vi "User data_MClr.vi"(0 "Inspector":string="ID-0", 1 "Station":string="EQD", 2 "Vendor":string="Icon", 3 "Number":string="?", 4 "PO#":string="?", 5 "Error In":errorcluster, 6 "base path":path=path "C:/", 8 "prompt (Create Folder)":string="logsController", 10 "file name":string) -> (14 "refnum out":refnum<file>, 19 "error out":errorcluster)   [LabVIEW 2018]
uses:
  Global textParse.vi
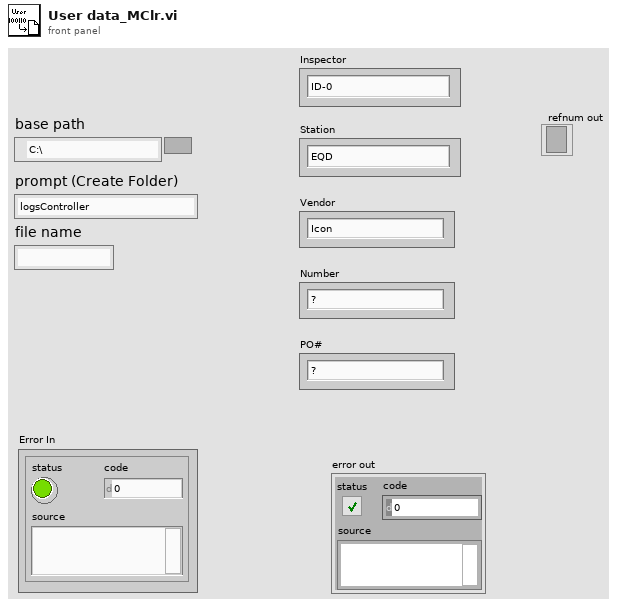
[diagram p1: front panel]
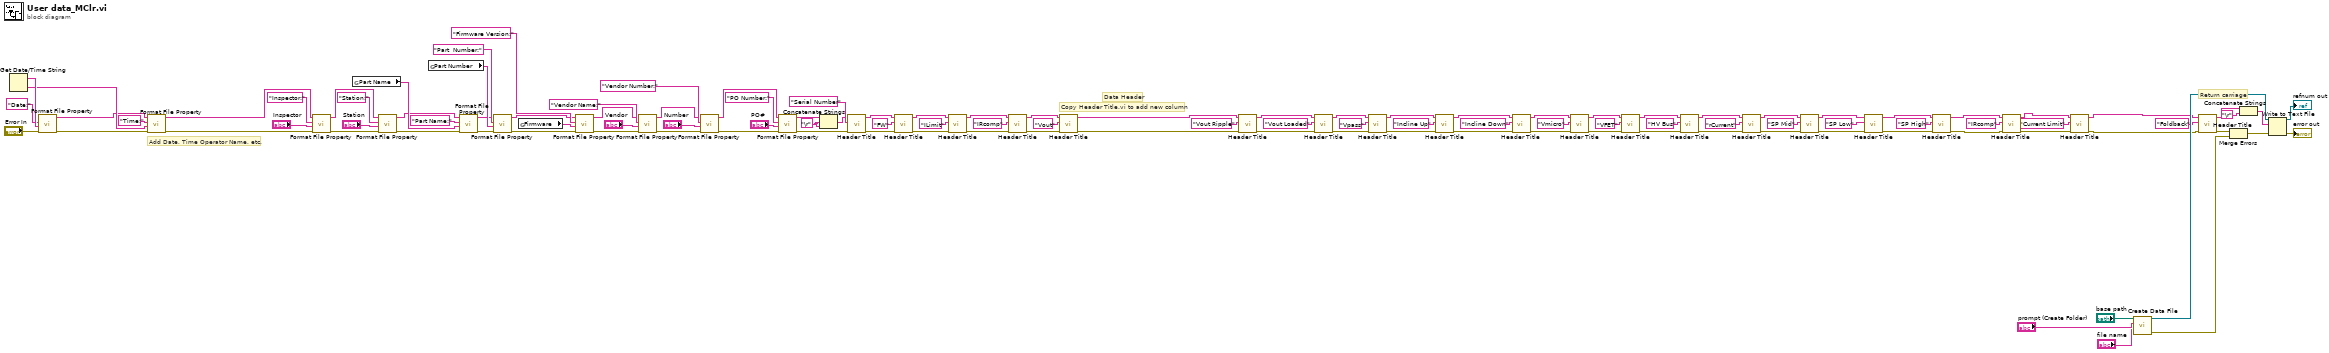
[diagram p0: block diagram]
diagram:
  w74 = "\r"
  # "Return carriage"
  # "Copy Header Title.vi to add new column"
  # "Data Header"
  # "Add Date, Time Operator Name, etc."
  n1 = Get Date/Time String() -> (date string=w110:string, time string=w101:string)  [unwired: 3 in]
  n2 = call "Format File Property.vi"("Error In"="Error In", "File Property Value"=w110, "File Property Name"="Date:") -> ("Error Out"=w108:errorcluster, "String out"=w36:string)  [unwired: 7 in]
  n3 = call "Format File Property.vi"("Error In"=w108, "File Property Value"=w101, "File Property Name"="Time:", "String in"=w36) -> ("Error Out"=w109:errorcluster, "String out"=w35:string)  [unwired: 6 in]
  n4 = call "Format File Property.vi"("Error In"=w109, "File Property Value"="Inspector", "File Property Name"="Inspector:", "String in"=w35) -> ("Error Out"=w107:errorcluster, "String out"=w34:string)  [unwired: 6 in]
  n5 = global read "Global textParse.vi" "Part Name"() -> (w98:string)
  n6 = call "Format File Property.vi"("Error In"=w107, "File Property Value"="Station", "File Property Name"="Station:", "String in"=w34) -> ("Error Out"=w100:errorcluster, "String out"=w33:string)  [unwired: 6 in]
  n7 = global read "Global textParse.vi" "Part Number"() -> (w112:string)
  n8 = call "Format File Property.vi"("Error In"=w100, "File Property Value"=w98, "File Property Name"="Part Name:", "String in"=w33) -> ("Error Out"=w99:errorcluster, "String out"=w32:string)  [unwired: 6 in]
  n9 = call "Format File Property.vi"("Error In"=w99, "File Property Value"=w112, "File Property Name"="Part  Number:", "String in"=w32) -> ("Error Out"=w111:errorcluster, "String out"=w31:string)  [unwired: 6 in]
  n10 = global read "Global textParse.vi" "Firmware"() -> (w113:string)
  n11 = call "Format File Property.vi"("Error In"=w111, "File Property Value"=w113, "File Property Name"="Firmware Version:", "String in"=w31) -> ("Error Out"=w9:errorcluster, "String out"=w12:string)  [unwired: 6 in]
  n12 = call "Format File Property.vi"("Error In"=w9, "File Property Value"="Vendor", "File Property Name"="Vendor Name:", "String in"=w12) -> ("Error Out"=w22:errorcluster, "String out"=w19:string)  [unwired: 6 in]
  n13 = call "Format File Property.vi"("Error In"=w22, "File Property Value"="Number", "File Property Name"="Vendor Number:", "String in"=w19) -> ("Error Out"=w13:errorcluster, "String out"=w14:string)  [unwired: 6 in]
  n14 = call "Format File Property.vi"("Error In"=w13, "File Property Value"="PO#", "File Property Name"="PO Number:", "String in"=w14) -> ("Error Out"=w10:errorcluster, "String out"=w11:string)  [unwired: 6 in]
  n15 = Concatenate Strings(w11, w74, w74) -> (w75:string)
  n16 = call "Header Title.vi"("Error In"=w10, "Header Title"="Serial Number" ("string"), "String in"=w75) -> ("Error Out"=w40:errorcluster, "String out"=w39:string)  [unwired: 7 in]
  n17 = call "Header Title.vi"("Error In"=w40, "Header Title"="FW", "String in"=w39) -> ("Error Out"=w47:errorcluster, "String out"=w46:string)  [unwired: 7 in]
  n18 = call "Header Title.vi"("Error In"=w47, "Header Title"="ILimit", "String in"=w46) -> ("Error Out"=w45:errorcluster, "String out"=w44:string)  [unwired: 7 in]
  n19 = call "Header Title.vi"("Error In"=w45, "Header Title"="IRcomp", "String in"=w44) -> ("Error Out"=w37:errorcluster, "String out"=w38:string)  [unwired: 7 in]
  n20 = call "Header Title.vi"("Error In"=w37, "Header Title"="Vout" ("string"), "String in"=w38) -> ("Error Out"=w77:errorcluster, "String out"=w81:string)  [unwired: 7 in]
  n21 = call "Header Title.vi"("Error In"=w77, "Header Title"="Vout Ripple" ("string"), "String in"=w81) -> ("Error Out"=w56:errorcluster, "String out"=w80:string)  [unwired: 7 in]
  n22 = call "Header Title.vi"("Error In"=w56, "Header Title"="Vout Loaded" ("string"), "String in"=w80) -> ("Error Out"=w52:errorcluster, "String out"=w55:string)  [unwired: 7 in]
  n23 = call "Header Title.vi"("Error In"=w52, "Header Title"="Vpass", "String in"=w55) -> ("Error Out"=w53:errorcluster, "String out"=w54:string)  [unwired: 7 in]
  n24 = call "Header Title.vi"("Error In"=w53, "Header Title"="Incline Up" ("Measured Data"), "String in"=w54) -> ("Error Out"=w51:errorcluster, "String out"=w79:string)  [unwired: 7 in]
  n25 = call "Header Title.vi"("Error In"=w51, "Header Title"="Incline Down" ("Measured Data"), "String in"=w79) -> ("Error Out"=w48:errorcluster, "String out"=w49:string)  [unwired: 7 in]
  n26 = call "Header Title.vi"("Error In"=w48, "Header Title"="Vmicro", "String in"=w49) -> ("Error Out"=w68:errorcluster, "String out"=w73:string)  [unwired: 7 in]
  n27 = call "Header Title.vi"("Error In"=w68, "Header Title"="VFET", "String in"=w73) -> ("Error Out"=w67:errorcluster, "String out"=w72:string)  [unwired: 7 in]
  n28 = call "Header Title.vi"("Error In"=w67, "Header Title"="HV Bus", "String in"=w72) -> ("Error Out"=w66:errorcluster, "String out"=w71:string)  [unwired: 7 in]
  n29 = call "Header Title.vi"("Error In"=w66, "Header Title"="rCurrent", "String in"=w71) -> ("Error Out"=w26:errorcluster, "String out"=w27:string)  [unwired: 7 in]
  n30 = call "Header Title.vi"("Error In"=w26, "Header Title"="SP Mid", "String in"=w27) -> ("Error Out"=w65:errorcluster, "String out"=w70:string)  [unwired: 7 in]
  n31 = call "Header Title.vi"("Error In"=w65, "Header Title"="SP Low", "String in"=w70) -> ("Error Out"=w64:errorcluster, "String out"=w69:string)  [unwired: 7 in]
  n32 = call "Header Title.vi"("Error In"=w64, "Header Title"="SP High", "String in"=w69) -> ("Error Out"=w3:errorcluster, "String out"=w4:string)  [unwired: 7 in]
  n33 = call "Header Title.vi"("Error In"=w3, "Header Title"="IRcomp", "String in"=w4) -> ("Error Out"=w2:errorcluster, "String out"=w5:string)  [unwired: 7 in]
  n34 = call "Header Title.vi"("Error In"=w2, "Header Title"="Current Limit", "String in"=w5) -> ("Error Out"=w1:errorcluster, "String out"=w6:string)  [unwired: 7 in]
  n35 = call "Create Data File.vi"("file name"="file name", "prompt (Create Folder)"="prompt (Create Folder)", "base path"="base path") -> ("Error Out"=w102:errorcluster, "File Refnum"=w104:refnum<file>)  [unwired: 7 in]
  n36 = call "Header Title.vi"("Error In"=w1, "Header Title"="Foldback", "String in"=w6) -> ("Error Out"=w29:errorcluster, "String out"=w30:string)  [unwired: 7 in]
  n37 = Merge Errors(w29, w102) -> (w103:errorcluster)
  n38 = Concatenate Strings(w30, "\r") -> (w76:string)
  n39 = Write to Text File(file (use dialog)=w104, text=w76, error in=w103) -> (refnum out=→"refnum out":refnum<file>, error out=→"error out":errorcluster)  [unwired: 1 in, 1 out]
